vi "Serial_Port_FGV.vi"(8 "error in (no error)":errorcluster, 9 "Initialize ?":bool, 10 "baud rate":u32=9600, 11 "COM Port In":refnum<visa-resource-name>) -> (0 "error out":errorcluster, 3 "COM Port out":refnum<visa-resource-name>)   [LabVIEW 2017]
uses:
  <vilib>/Instr/_visa.llb/VISA Configure Serial Port (Instr).vi
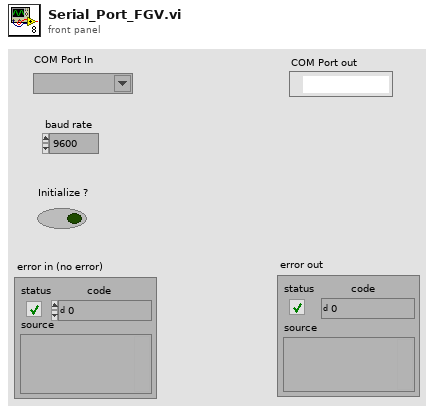
[diagram p1: front panel]
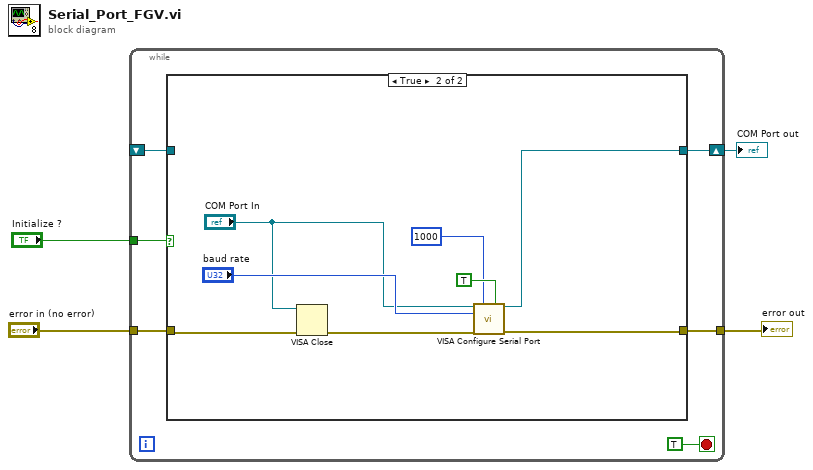
[diagram p0: block diagram]
diagram:
  n1 = while {
    tunnel: "error in (no error)" -> [w10]
    tunnel: "Initialize ?" -> [w9]
    tunnel: [w8] -> w2
    shift-right: [w7] -> w1
    shift-left: _ -> [w6]
    stop <- TRUE stop-if-true
    n2 = case shown="True" w9 {
      tunnel: w10 -> [w11 w16]
      tunnel: [w11 w20] -> w8
      tunnel: [w12 w18] -> w7
      tunnel: w6 -> [w12 _]
      frame False {
      }
      frame True {
        n3 = VISA Close(VISA resource name="COM Port In", error in (no error)=w16) -> (error out=w14:errorcluster)
        n4 = call-poly "VISA Configure Serial Port"("VISA resource name"="COM Port In", "timeout (10sec)"=u32 1000, "Enable Termination\nChar (T)"=TRUE ("Enable Termination\nChar (T)"), "baud rate (9600)"="baud rate", "error in (no error)"=w14) -> ("VISA resource name out"=w18:refnum<visa-resource-name>, "error out"=w20:errorcluster)  [unwired: 9 in]
      }
    }
  }
  "error out" <- w2
  "COM Port out" <- w1
